vi "Method.vi"(4 "B":refnum<class "Abs_Integer.lvclass">, 5 "A":T1) -> (1 "Result":T1)   [LabVIEW 2021, in "EXOR_U16.lvclass"]
uses:
  EXOR_U16.lvclass
  Abs_Type.ctl
  Abs_Types/U16 Integer/Abs_U16 Integer.lvclass
  Abs_Types/Integer/Abs_Integer.lvclass
  C:/Program Files (x86)/National Instruments/LabVIEW 2021/vi.lib/TSA/Abstract Data Classes/Abs_Types/Numeric/Abs_Numeric.lvclass
  C:/TSA/LV_Abstract/Source/Functions/Support/Function/Two Terminal/U16/AbsFunc_Two Term_U16.lvclass
  C:/Program Files (x86)/National Instruments/LabVIEW 2021/vi.lib/TSA/Abstract Data Classes/Abs_Types/U16 Integer/Abs_U16 Integer.lvclass
  Support/Function/Two Terminal/U16/AbsFunc_Two Term_U16.lvclass/AbsFunc_Two Term_U16.ctl
  Support/Function/Two Terminal/U16/Properties/Write Numeric A.vi
  Support/Function/Two Terminal/U16/Properties/Write Numeric B.vi
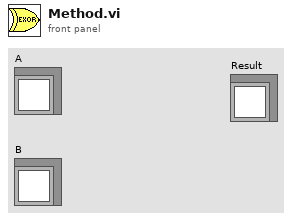
[diagram p1: front panel]
types:
  T1 = typedef "EXOR_U16.lvclass/Abs_Type.ctl" = refnum<class "Abs_U16 Integer.lvclass">
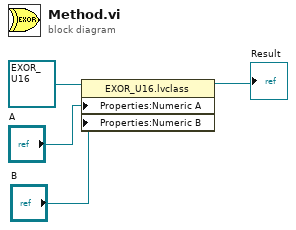
[diagram p0: block diagram]
diagram:
  n1 = property class="EXOR_U16.lvclass"(reference=refnum<class "EXOR_U16.lvclass"> refnum ("Functions.lvlib:Logic.lvlib:AND.lvclass"), "Properties:Numeric A"="A", "Properties:Numeric B"="B") -> (reference out=→"Result":refnum<class "EXOR_U16.lvclass">)  [unwired: 1 in, 1 out]
